vi "test Inner Handle Method.vi"(8 "error in (no error)":errorcluster, 11 "TestCase in":refnum<class "Memory Manager Tests.lvclass">) -> (0 "error out":errorcluster, 3 "TestCase out":refnum<class "Memory Manager Tests.lvclass">)   [LabVIEW 2020, in "Memory Manager Tests.lvclass"]
uses:
  Memory Manager Tests.lvclass
  Memory Manager Tests.lvclass/Memory Manager Tests.ctl
  <vilib>/addons/_JKI Toolkits/VI Tester/TestCase.llb/TestCase.lvclass
  C:/Program Files/National Instruments/LabVIEW 2020/vi.lib/addons/_JKI Toolkits/VI Tester/TestCase.llb/TestCase.lvclass
panel:
  out "return type":i32
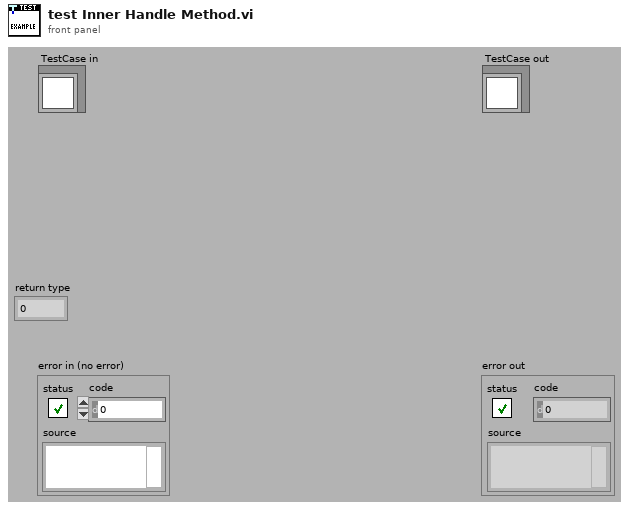
[diagram p1: front panel]
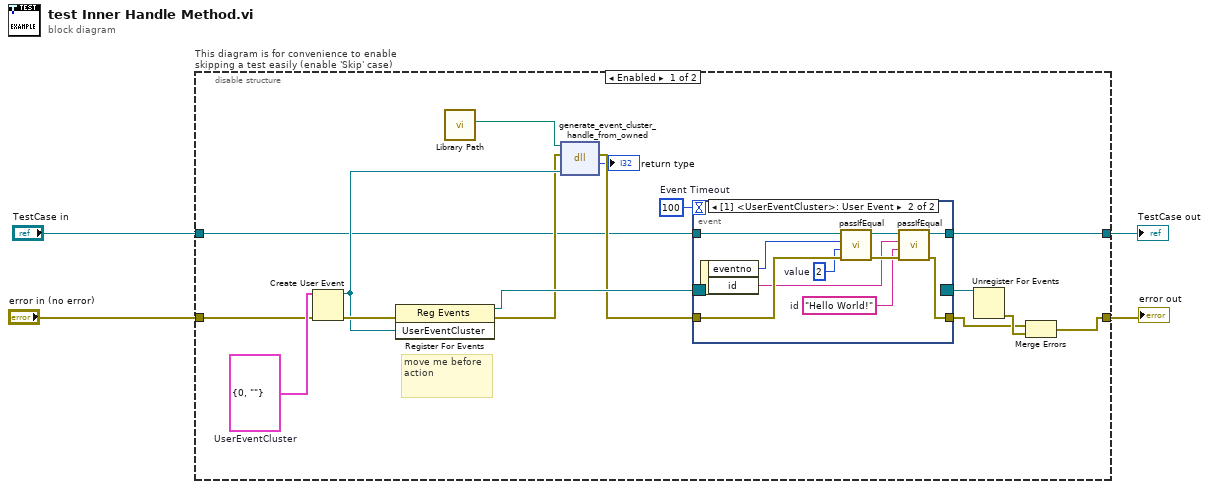
[diagram p0: block diagram]
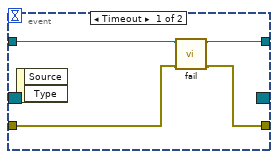
[diagram p2: hidden frame]
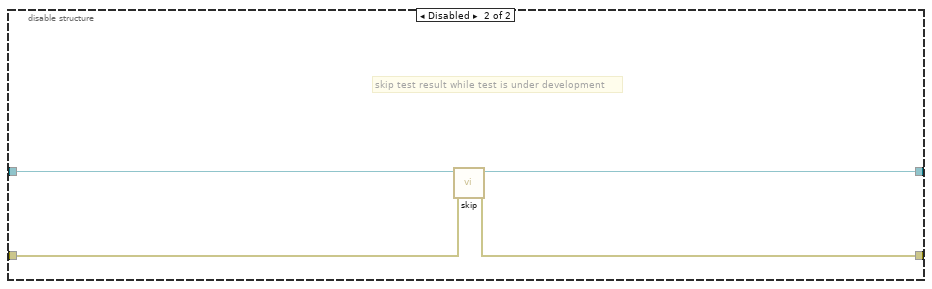
[diagram p3: hidden frame]
diagram:
  n1 = disable-structure "This diagram is for convenience to enable skipping a test easily (enable 'Skip' case)" shown="Enabled" {
    disable-tunnel: "TestCase in" -> [w8 w38]
    disable-tunnel: [w7 w36] -> w1
    disable-tunnel: [w6 w37] -> w3
    disable-tunnel: "error in (no error)" -> [w5 w35]
    frame Enabled {
      w9 = cluster{"eventno":i32, "id":string} {"eventno"=0, "id"=""}  # UserEventCluster
      w16 = 100  # Event Timeout
      # "move me before\naction"
      n2 = Create User Event(user event datatype=w9, error in=w5) -> (user event=w13:refnum<user-event>, error out=w15:errorcluster)
      n3 = register-events(error in=w15, w13) -> (reference out=w20:refnum<event-registration>, error out=w12:errorcluster)  [unwired: 1 in]
      n4 = call "Library Path.vi"() -> ("Library Path"=w14:path)  [unwired: 11 in]
      n5 = dll-call lib="C:/Users/JamesMcNally/Documents/RustInterop/Rust-LabVIEW-Interop/target/debug/labview_test_library.dll" fn="generate_event_cluster_handle_from_owned"(path in=w14, error in=w12, "event"=w13) -> (error out=w11:errorcluster, "return type"=→"return type":i32)  [unwired: 2 in, 1 out]
      n6 = event shown="[1] <UserEventCluster>: User Event" {
        selector: w20 -> [_ _]
        dyn-events: [_ _] -> w17
        timeout: w16 -> [_ _]
        tunnel: w8 -> [w24 w34]
        tunnel: [w23 w27] -> w7
        tunnel: [w21 w29] -> w18
        tunnel: w11 -> [w22 w32]
        event Timeout {
          n7 = event-data() -> ()  [unwired: 1 in, 2 out]
          n8 = call-dynamic "fail.vi"("error in (no error)"=w22, "TestCase in"=w24) -> ("error out"=w21:errorcluster, "TestCase out"=w23:refnum<class "Memory Manager Tests.lvclass">)  [unwired: 8 in]
        }
        event User Event {
          w25 = "Hello World!"  # id
          w31 = 2  # value
          n9 = event-data() -> ("eventno"=w30:i32, "id"=w26:string)  [unwired: 1 in]
          n10 = call-dynamic "passIfEqual.vi"("error in (no error)"=w32, "y"=w31, "x"=w30, "TestCase in"=w34) -> ("error out"=w33:errorcluster, "TestCase out"=w28:refnum<class "Memory Manager Tests.lvclass">)  [unwired: 6 in]
          n11 = call-dynamic "passIfEqual.vi"("error in (no error)"=w33, "y"=w25, "x"=w26, "TestCase in"=w28) -> ("error out"=w29:errorcluster, "TestCase out"=w27:refnum<class "Memory Manager Tests.lvclass">)  [unwired: 6 in]
        }
      }
      n12 = Unregister For Events(event registration refnum=w17) -> (error out=w19:errorcluster)  [unwired: 1 in]
      n13 = Merge Errors(w18, w19) -> (w6:errorcluster)
    }
    frame Disabled {
      # "skip test result while test is under development"
      n14 = call <vilib>:"skip.vi"("error in (no error)"=w35, "TestCase in"=w38) -> ("error out"=w37:errorcluster, "TestCase out"=w36:refnum<class "Memory Manager Tests.lvclass">)  [unwired: 8 in]
    }
  }
  "error out" <- w3
  "TestCase out" <- w1
